vi "BRig_Host__Loop_Producer__tcp_System__Data_prepareFilepaths_source__v2.vi"(8 "input_arrFilenames":string[](array[string]), 9 "input_nFilenames":i32, 11 "input_expPrefix":string) -> (3 "output_arrPath":path[](array[path]))   [LabVIEW 2014]
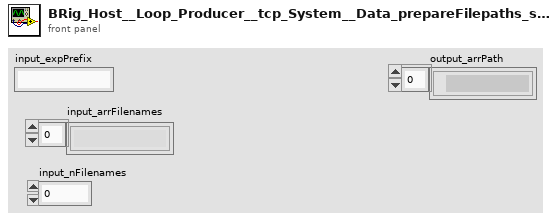
[diagram p1: front panel]
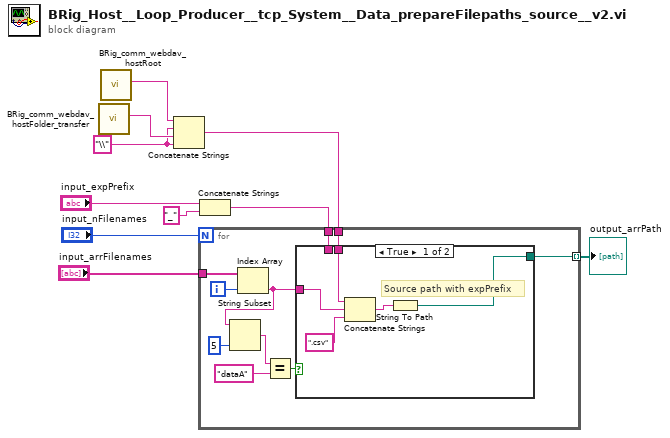
[diagram p0: block diagram]
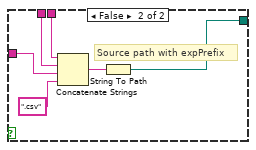
[diagram p2: hidden frame]
diagram:
  w4 = "\\" ("string")
  n1 = call "BRig_comm_webdav_hostFolder_transfer.vi"() -> ("output_HostFolder"=w5:string)  [unwired: 11 in]
  n2 = call "BRig_comm_webdav_hostRoot.vi"() -> ("output_hostRoot"=w3:string)  [unwired: 11 in]
  n3 = Concatenate Strings(w3, w4, w5, w4) -> (w2:string)
  n4 = Concatenate Strings("input_expPrefix", "_" ("string")) -> (w7:string)
  n5 = for {
    N: "input_nFilenames" -> [_]
    tunnel: w7 -> [w17]
    tunnel: "input_arrFilenames" -> [w20]
    tunnel: w2 -> [w18]
    tunnel: [w16] -> w1 mode=indexing
    i -> [w19]
    n6 = Index Array(array=w20, index=w19) -> (element=w15:string)
    n7 = String Subset(string=w15, length (rest)=5 ("length (rest)")) -> (substring=w13:string)  [unwired: 1 in]
    n8 = Equal?(x=w13, y="dataA") -> (x = y?=w11:bool)
    n9 = case shown="True" w11 {
      tunnel: w18 -> [w21 w30]
      tunnel: w17 -> [_ w29]
      tunnel: [w23 w27] -> w16
      tunnel: w15 -> [w22 w26]
      frame True {
        # "Source path with expPrefix"
        n10 = Concatenate Strings(w21, w22, ".csv" ("string")) -> (w25:string)
        n11 = String To Path(string=w25) -> (path=w23:path)
      }
      frame False {
        # "Source path with expPrefix"
        n12 = Concatenate Strings(w30, w29, w26, ".csv" ("string")) -> (w31:string)
        n13 = String To Path(string=w31) -> (path=w27:path)
      }
    }
  }
  "output_arrPath" <- w1
